vi "GET SV Variables from Target.vi"(7 "Read/Write":string, 8 "error in (no error)":errorcluster, 11 "Target":string) -> (0 "error out":errorcluster, 3 "Channel Array":refnum<class "ChannelVS.lvclass">[](array[class]))   [LabVIEW 2017, in "Shared Variables CD 2.0 Configuration.lvlib"]
uses:
  Shared Variables CD 2.0 Configuration.lvlib
  ChannelVS/ChannelVS.lvclass
  IPAddress Functions/ValidIPAddr.vi
  <vilib>/Utility/error.llb/Error Cluster From Error Code.vi
  Shared/SV Global.vi
  <resource>/objmgr/ni.var.rc
  Public/Documents/National Instruments/NI VeriStand 2017/Custom Devices/Shared Variables CD 2.0/Data/Channel.lvlibp/Channel.lvclass
  <vilib>/Utility/Data Type/NI_Data Type.lvlib
  C:/Users/Public/Documents/National Instruments/NI VeriStand 2017/Custom Devices/Shared Variables CD 2.0/Data/Channel.lvlibp/Channel.lvclass
panel:
  # "Loading....."
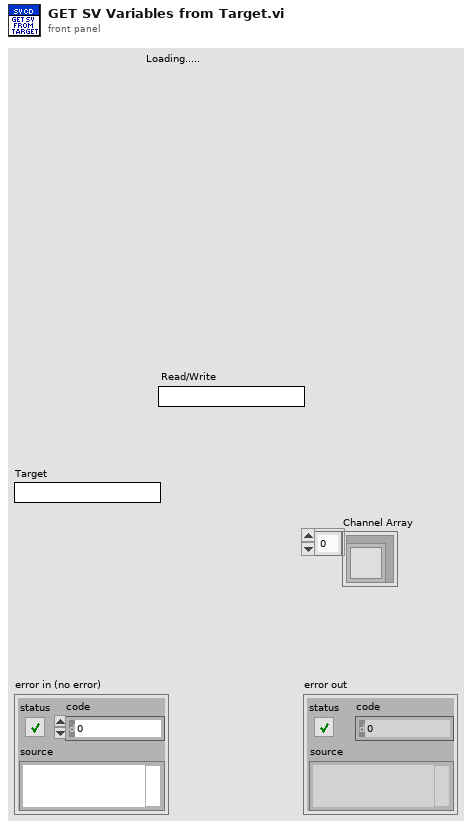
[diagram p1: front panel]
types:
  T1 = typedef "NI_Data Type.lvlib/Data Type.ctl" = enum8{"Invalid Type", "Void", "I8", "I16", "I32", "I64", "U8", "U16", "U32", "U64", "Single Float", "Double Float", "Extended Float", "Single Complex", "Double Complex", "Extended Complex", "Enum U8", "Enum U16", "Enum U32", "Enum U64", "Single Float With Unit", "Double Float With Unit", "Extended Float With Unit", "Single Complex with Unit", "Double Complex with Unit", "Extended Complex with Unit", "Boolean", "String", "Path", "Picture", "Tag", "Array", "Cluster", "Variant", "LV Variant", "Waveform", "Timestamp", "Digital Waveform", "Digital Data", "ExpressData", "Refnum", "External Data", "VI", "Poly VI", "LabVIEW Class Instance", "Fixed Point"}
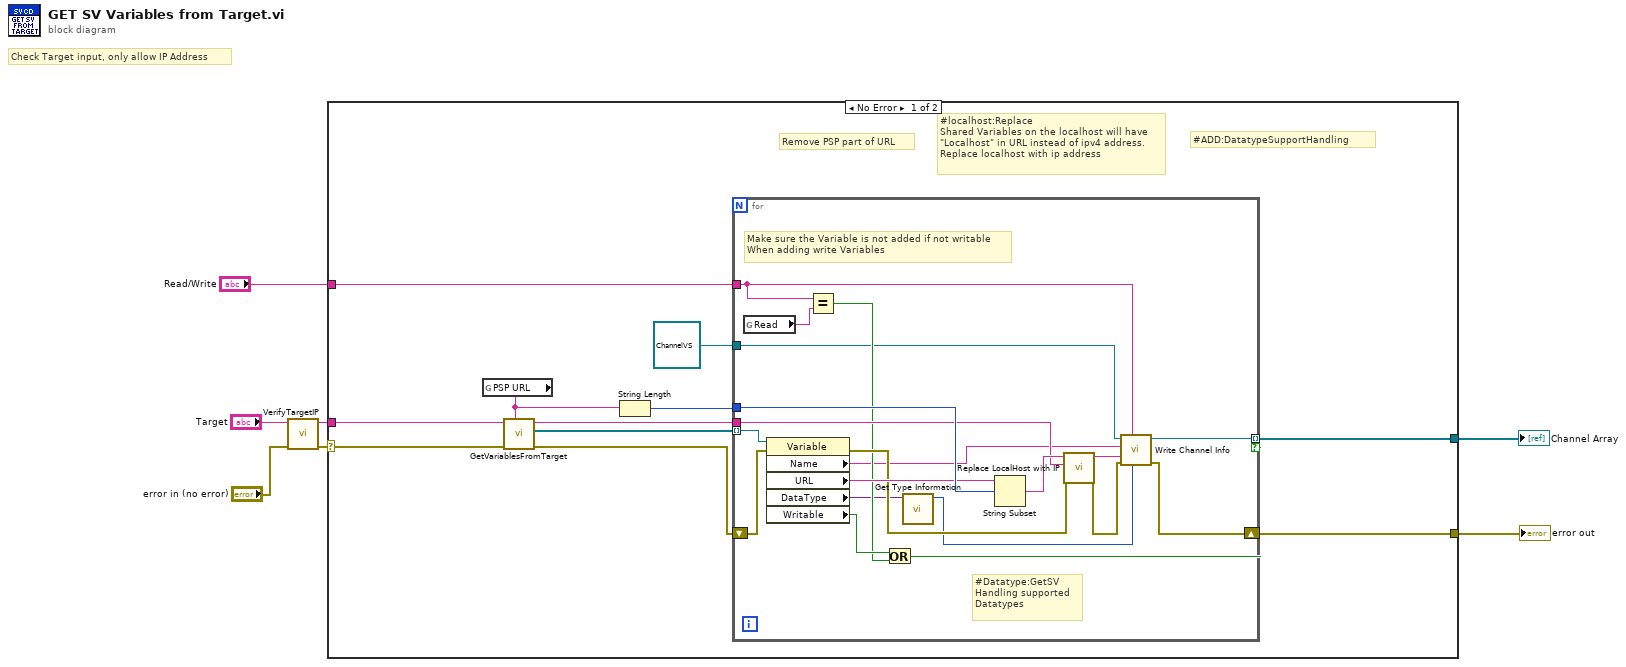
[diagram p0: block diagram]
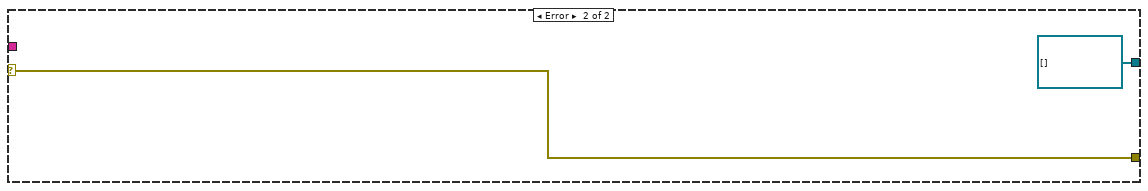
[diagram p2: hidden frame]
diagram:
  # "Check Target input, only allow IP Address"
  n1 = call "VerifyTargetIP.vi"("error in (no error)"="error in (no error)", "Target"="Target") -> ("error out"=w4:errorcluster, "IP Address String out"=w3:string)  [unwired: 8 in]
  n2 = case shown="No Error" w4 {
    selector: w4 -> [w10 w40]
    tunnel: w3 -> [w14 _]
    tunnel: [w17 w40] -> w7
    tunnel: [w16 refnum<class "ChannelVS.lvclass">[] []] -> w1
    tunnel: "Read/Write" -> [w9 _]
    frame No Error {
      # "#ADD:DatatypeSupportHandling"
      # "#localhost:Replace\nShared Variables on the localhost will have\n\"Localhost\" in URL instead of ipv4 address.\nReplace localhost with ip address"
      # "Remove PSP part of URL"
      n3 = global read "SV Global.vi" "PSP URL"() -> (w11:string)
      n4 = call "GetVariablesFromTarget.vi"("PSP URL(ni.var.psp://)"=w11, "error in (no error)"=w10, "IP Address String in"=w14) -> ("error out"=w18:errorcluster, "AllVariables[]"=w13:refnum<k21>[], "IP Address String out"=w12:string)  [unwired: 6 in]
      n5 = String Length(string=w11) -> (length=w15:i32)
      n6 = for {
        shift-right: [w25] -> w17
        shift-left: w18 -> [w38]
        tunnel: [w19] -> w16 mode=indexing if=w22
        tunnel: w15 -> [w37]
        tunnel: w13 -> [w33] mode=indexing
        tunnel: w12 -> [w32]
        tunnel: w9 -> [w24]
        tunnel: refnum<class "ChannelVS.lvclass"> refnum ("Shared Variables CD 2.0 Configuration.lvlib:ChannelVS.lvclass") -> [w23]
        # "Make sure the Variable is not added if not writable\nWhen adding write Variables"
        # "#Datatype:GetSV\nHandling supported\nDatatypes"
        n7 = global read "SV Global.vi" "Read"() -> (w30:string)
        n8 = property class="Variable"(reference=w33, error in=w38) -> (error out=w34:errorcluster, "Name"=w27:string, "URL"=w36:string, "DataType"=w21:variant, "Writable"=w31:bool)  [unwired: 1 out]
        n9 = Equal?(x=w24, y=w30) -> (x = y?=w29:bool)
        n10 = Or(x=w31, y=w29) -> (x .or. y?=w22:bool)
        n11 = call <vilib>:"Get Type Information.vi"("Variant"=w21) -> ("Type"=w20:T1)  [unwired: 6 in, 4 out]
        n12 = String Subset(string=w36, offset (0)=w37) -> (substring=w35:string)  [unwired: 1 in]
        n13 = call "Replace LocalHost with IP.vi"("error in (no error)"=w34, "IP Address"=w32, "URL"=w35) -> ("error out"=w26:errorcluster, "URL with IP"=w28:string)  [unwired: 7 in]
        n14 = call "Write Channel Info.vi"("DataType"=w20, "Read or Write"=w24, "error in (no error)"=w26, "URL"=w28, "Name"=w27, "Channel in"=w23) -> ("error out"=w25:errorcluster, "Channel out"=w19:refnum<class "ChannelVS.lvclass">)  [unwired: 4 in]
      }
    }
    frame Error {
    }
  }
  "error out" <- w7
  "Channel Array" <- w1
